vi "processNodes.vi"(8 "error in (no error)":errorcluster, 9 "Calling VI Reference i":refnum<vi>, 10 "Nodes[]":refnum<vi>[](array[refnum]), 11 "VI in":refnum<class "VI.lvclass">) -> (0 "error out":errorcluster, 3 "VI out":refnum<class "VI.lvclass">)   [LabVIEW 2016, in "VI.lvclass"]
uses:
  VI.lvclass
  C:/LSST_TS/SystemSW/ct_tools/ProjectItem/ProjectItem.lvclass
  ProjectItem/ProjectItem.lvclass/ProjectItem.ctl
  Search/Search.lvclass/Search.ctl
  Node/Node.lvclass/Node.ctl
  INodeFactory/INodeFactory.lvclass
  Node/Node.lvclass
  Project/Project.lvclass
  Search/Search.lvclass
  ProjectItem/ProjectItem.lvclass
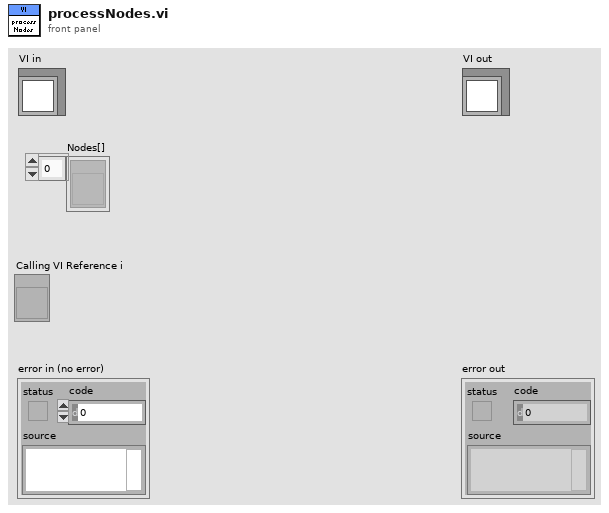
[diagram p1: front panel]
types:
  T1 = typedef "NodeSelection.ctl" = enum16{"Default", "CaseStructure", "EventStructure", "FlatSequence", "ForLoop", "WhileLoop"}
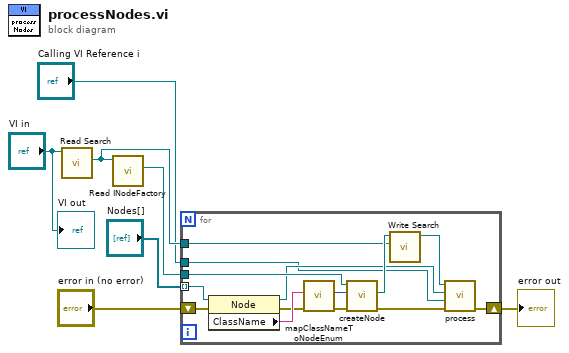
[diagram p0: block diagram]
diagram:
  n1 = call "Read Search.vi"("ProjectItem in"="VI in") -> ("Search"=w6:refnum<class "Search.lvclass">)  [unwired: 9 in, 1 out]
  n2 = call "Read INodeFactory.vi"("Search in"=w6) -> ("INodeFactory.lvclass"=w7:refnum<class "INodeFactory.lvclass">)  [unwired: 9 in, 1 out]
  n3 = for {
    tunnel: "Nodes[]" -> [w21] mode=indexing
    tunnel: w6 -> [w17]
    tunnel: w7 -> [w15]
    shift-right: [w10] -> w4
    shift-left: "error in (no error)" -> [w14]
    tunnel: "Calling VI Reference i" -> [w8]
    n4 = property class="Node"(reference=w21, error in=w14) -> (reference out=w9:refnum<vi>, error out=w13:errorcluster, "ClassName"=w20:string)
    n5 = call "mapClassNameToNodeEnum.vi"("error in (no error)"=w13, "Class Name"=w20) -> ("error out"=w12:errorcluster, "NodeSelection"=w19:T1)  [unwired: 7 in, 1 out]
    n6 = call-dynamic "createNode.vi"("error in (no error)"=w12, "NodeSelection"=w19, "INodeFactory in"=w15) -> ("error out"=w11:errorcluster, "Node"=w18:refnum<class "Node.lvclass">)  [unwired: 6 in, 1 out]
    n7 = call "Write Search.vi"("Search"=w17, "Node in"=w18) -> ("Node out"=w16:refnum<class "Node.lvclass">)  [unwired: 9 in]
    n8 = call-dynamic "process.vi"("error in (no error)"=w11, "Calling VI Reference i"=w8, "Node Refnum"=w9, "Node in"=w16) -> ("error out"=w10:errorcluster)  [unwired: 6 in, 1 out]
  }
  "error out" <- w4
  "VI out" <- "VI in"
